vi "Test ListBox VI.vi"() -> ()   [LabVIEW 2011]
uses:
  Selectable ListBox xControl/ListBox XControl.xctl
panel:
  in  "Select None":bool
  in  "Get":bool
  out "Selected Items []":string[](array[string])
  out "Selected Index []":i32[](array[numeric])
  in  "Invert":bool
  in  "Select All":bool
  in  "ListBox XControl":string[](xcontrol)
  # "By \n       Samuel James\n       LabVIEW Champion\n       Certified LabVIEW Architect\n       Assistant Lead Engineer\n       Vestas Technology R&D Chennai, India"
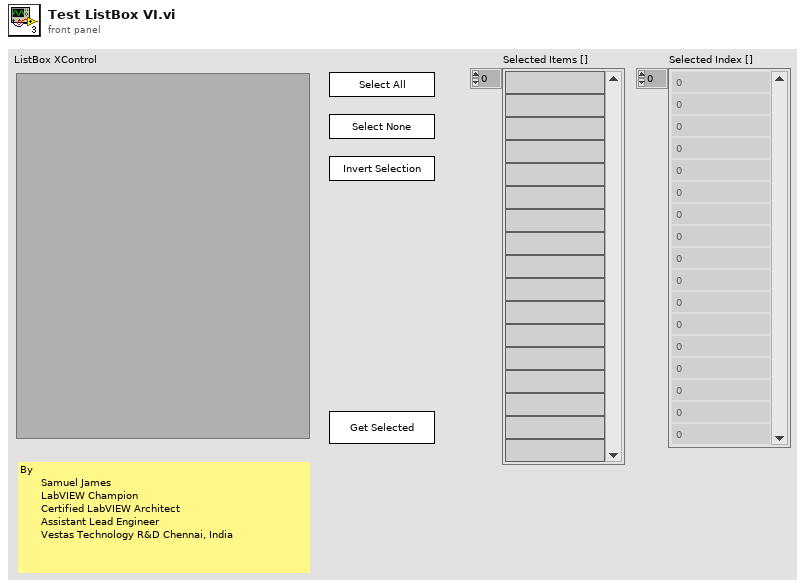
[diagram p1: front panel]
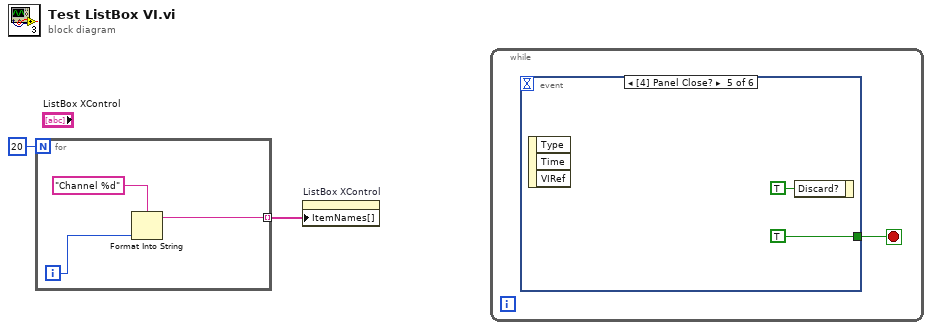
[diagram p0: block diagram]
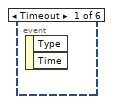
[diagram p2: hidden frame]
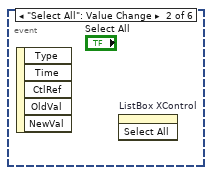
[diagram p3: hidden frame]
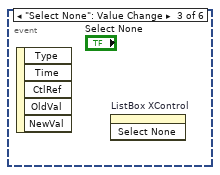
[diagram p4: hidden frame]
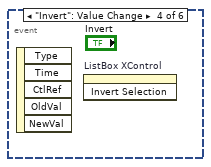
[diagram p5: hidden frame]
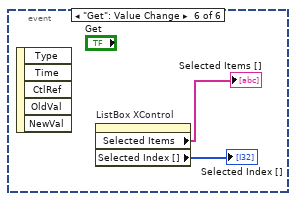
[diagram p6: hidden frame]
diagram:
  n1 = for {
    N: 20 -> [_]
    tunnel: [w3] -> w2 mode=indexing
    i -> [w5]
    n2 = Format Into String(format string="Channel %d", w5) -> (resulting string=w3:string)  [unwired: 2 in, 1 out]
  }
  n3 = property on="ListBox XControl" class="ListBox XControl (strict)"("ItemNames[]"=w2) -> ()  [unwired: 2 in, 2 out]
  n4 = while {
    stop <- w6 stop-if-true
    n5 = event shown="[4] Panel Close?" {
      selector: _ -> [_ _ _ _ _ _]
      dyn-events: _ -> [_ _ _ _ _ _]
      timeout: _ -> [_ _ _ _ _ _]
      tunnel: [_ _ _ _ TRUE _] -> w6
      event Timeout {
        n6 = event-data() -> ()  [unwired: 1 in, 2 out]
      }
      event "Select All": Value Change {
        n7 = event-data() -> ()  [unwired: 1 in, 5 out]
        n8 = invoke on="ListBox XControl" class="ListBox XControl (strict)" method="Select All"() -> ()  [unwired: 3 in, 3 out]
      }
      event "Select None": Value Change {
        n9 = event-data() -> ()  [unwired: 1 in, 5 out]
        n10 = invoke on="ListBox XControl" class="ListBox XControl (strict)" method="Select None"() -> ()  [unwired: 3 in, 3 out]
      }
      event "Invert": Value Change {
        n11 = event-data() -> ()  [unwired: 1 in, 5 out]
        n12 = invoke on="ListBox XControl" class="ListBox XControl (strict)" method="Invert Selection"() -> ()  [unwired: 3 in, 3 out]
      }
      event Panel Close? {
        n13 = event-data() -> ()  [unwired: 1 in, 3 out]
        n14 = event-data("Discard?"=TRUE) -> ()  [unwired: 1 in, 1 out]
      }
      event "Get": Value Change {
        n15 = event-data() -> ()  [unwired: 1 in, 5 out]
        n16 = property on="ListBox XControl" class="ListBox XControl (strict)"() -> ("Selected Items"=→"Selected Items []":string[], "Selected Index []"=→"Selected Index []":i32[])  [unwired: 2 in, 2 out]
      }
    }
  }
